vi "main_prototipo.vi"() -> ()   [LabVIEW 2021]
uses:
  Ctls/msg.ctl
  <vilib>/MakerHub/LINX/Private/Type Defs/LINX Ref.ctl
  <vilib>/MakerHub/LINX/Private/Type Defs/Platform.ctl
  <vilib>/MakerHub/LINX/Private/Type Defs/Interface.ctl
  <vilib>/MakerHub/LINX/Private/Device/Type Defs/LINX Device Config.ctl
  <vilib>/MakerHub/LINX/Private/Device/Type Defs/TCP Config.ctl
  <vilib>/MakerHub/LINX/Private/Device/Type Defs/Channels.ctl
  <vilib>/MakerHub/LINX/LMH-LINX.lvlib
  <vilib>/MakerHub/LINX/Private/Device/Device.lvlib
panel:
  in  "Stop":bool
  out "Datos Leídos":string[](array[string])
  in  "Buadrate":u32=8
  in  "Puerto COM":refnum<visa-resource-name>
  in  "TyP":bool
  out "Error Out 2":errorcluster
  in  "Error In 2":errorcluster
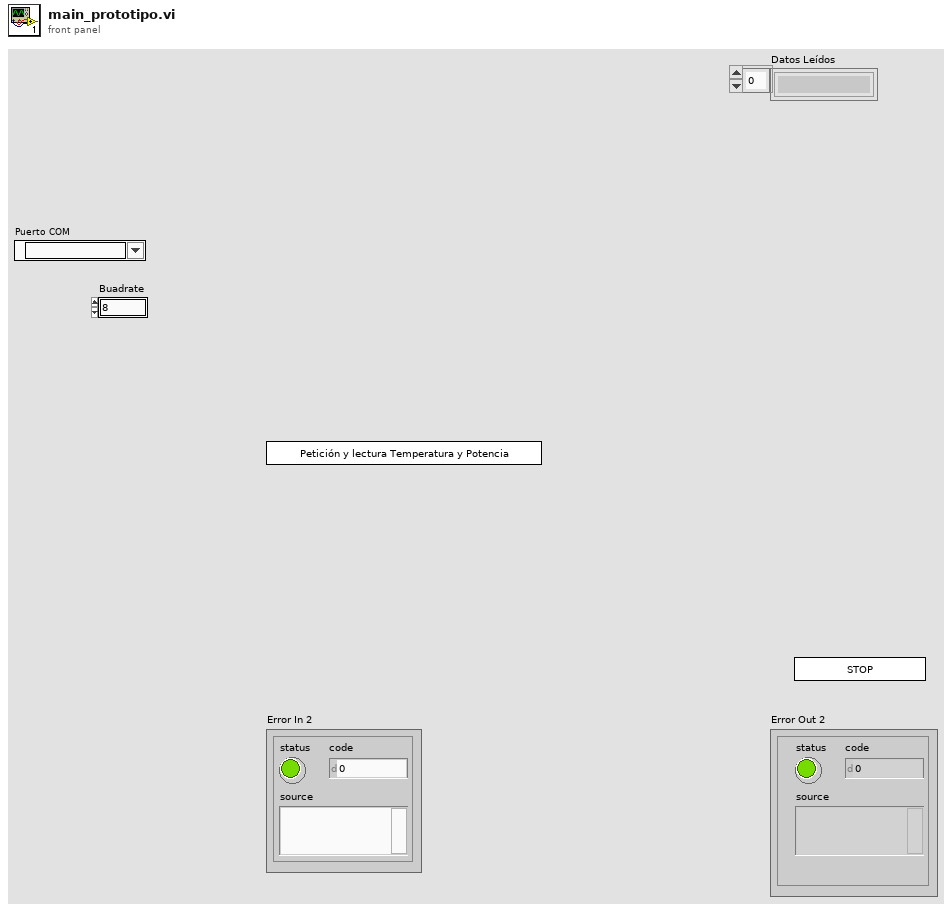
[diagram p1: front panel]
types:
  T1 = typedef "LMH-LINX.lvlib/LINX Ref.ctl" = cluster{"IO":T2, "Interface":T3, "LINX Device Config":T4}
  T2 = typedef "LMH-LINX.lvlib/Platform.ctl" = enum16{"Remote", "Local"}
  T3 = typedef "LMH-LINX.lvlib/Interface.ctl" = enum16{"Serial", "TCP"}
  T4 = typedef "LMH-LINX.lvlib/Device.lvlib/LINX Device Config.ctl" = cluster{"Interface":T3, "COM Port":refnum<visa-resource-name>, "TCP Configuration":T5, "Device Family":u8, "Device ID":u8, "Device Name":string, "TCP Ref":refnum<k5>, "Channels":T6}
  T5 = typedef "LMH-LINX.lvlib/Device.lvlib/TCP Config.ctl" = cluster{"IP Address":string, "Port":u16}
  T6 = typedef "LMH-LINX.lvlib/Channels.ctl" = cluster{"DI":u8[], "DO":u8[], "AI":u8[], "AO":u8[], "PWM":u8[], "QE":u8[], "UART":u8[], "I2C 2":u8[], "SPI":u8[], "CAN":u8[], "Servo":u8[], "AI Ref (V)":dbl, "AI Resolution (Bits)":u8, "AO Ref (V)":dbl, "AO Resolution (Bits)":u8}
  T7 = typedef "msg.ctl" = cluster{"mensaje":string, "info":cluster{"I2C Slave Address ":u8, "Data":u8[], "Bytes To Read":u8}, "LINX Resource":T1}
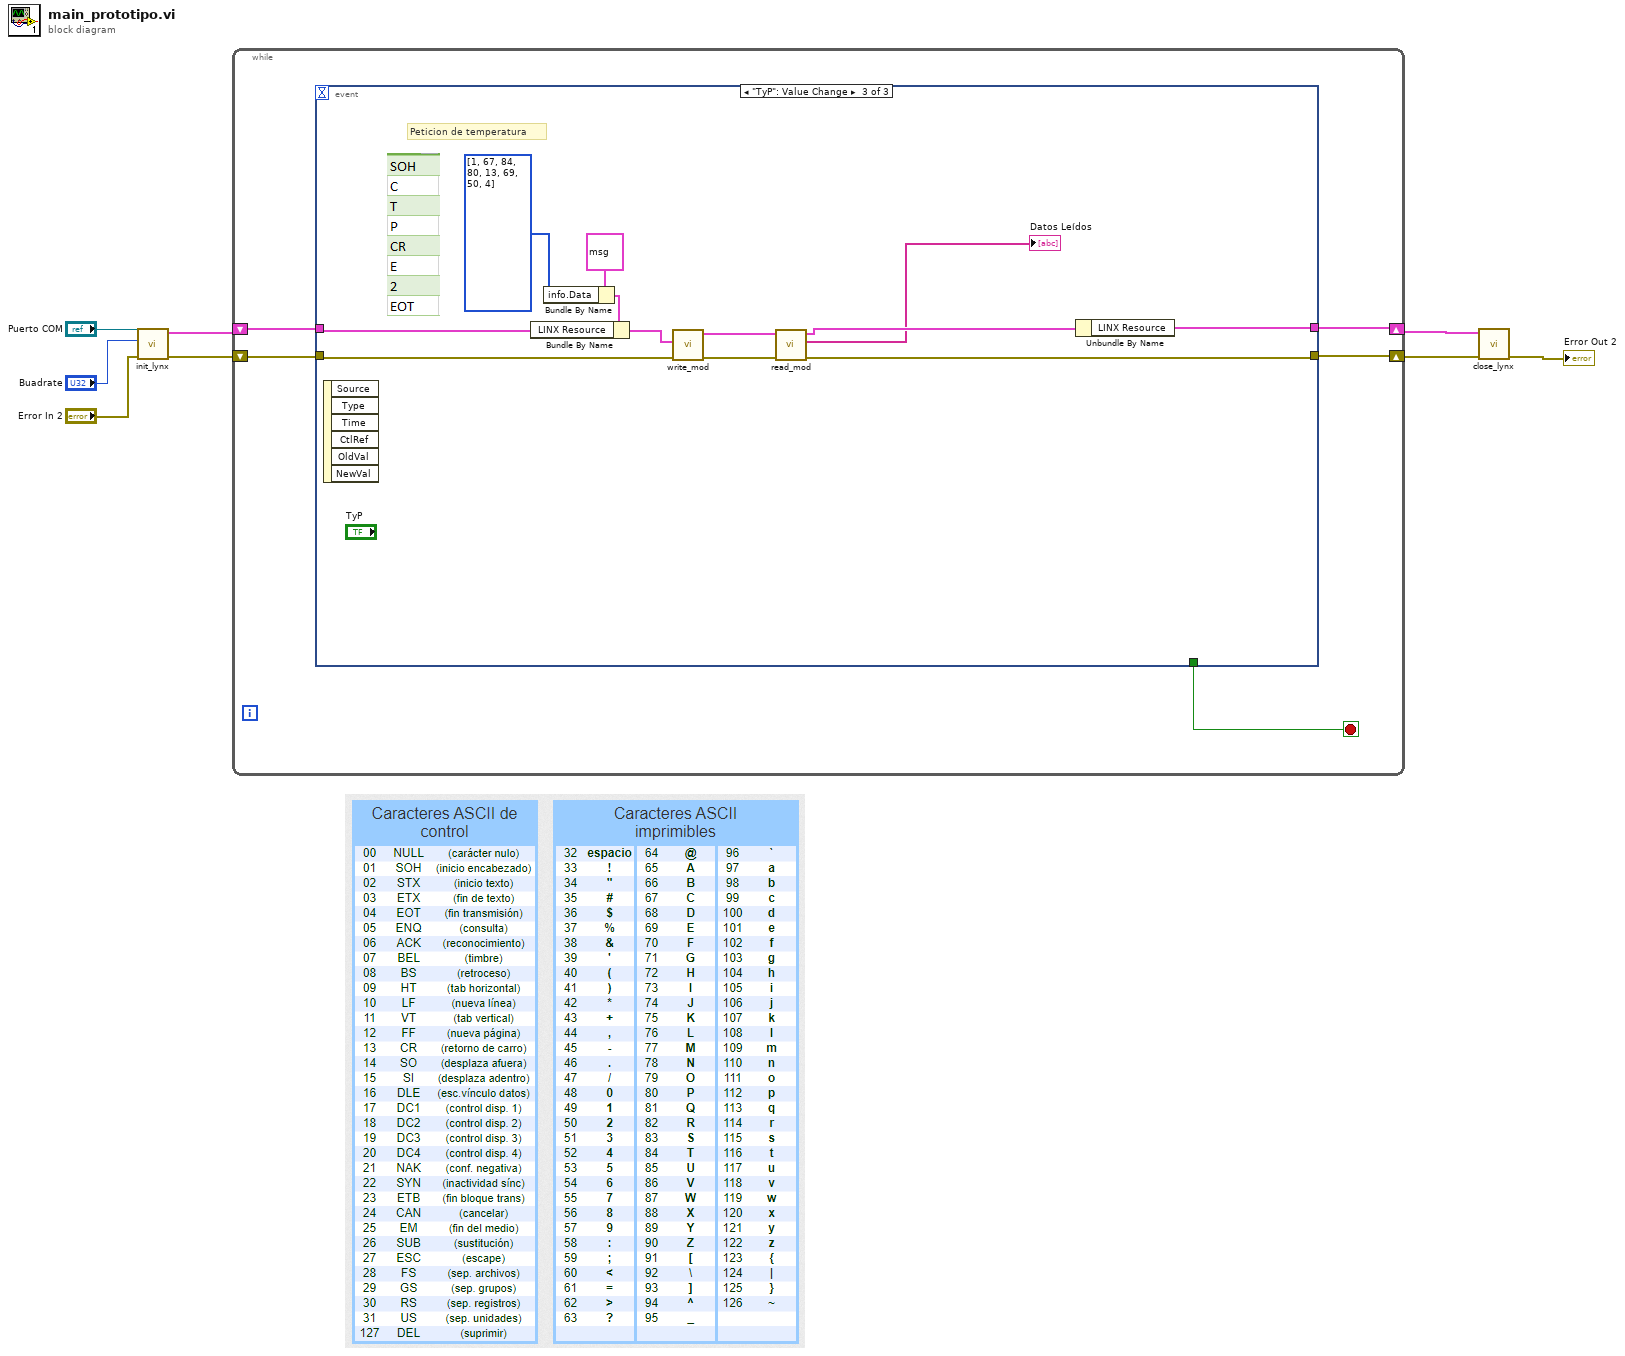
[diagram p0: block diagram]
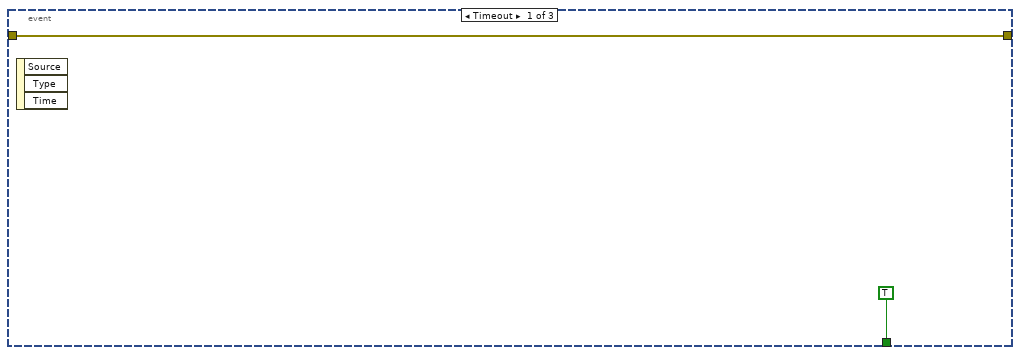
[diagram p2: hidden frame]
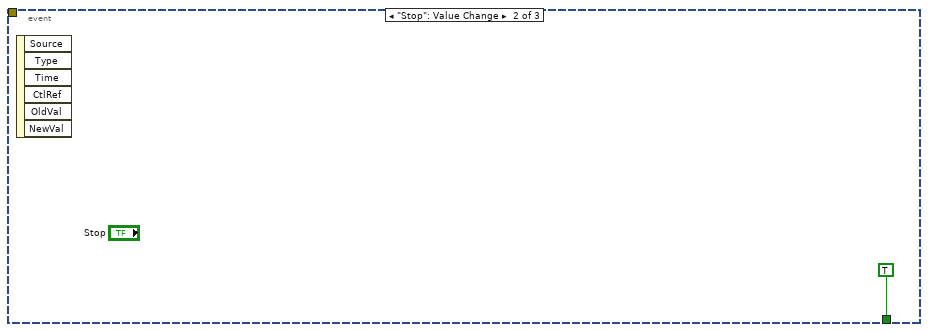
[diagram p3: hidden frame]
diagram:
  n1 = call "init_lynx.vi"("Error In 2"="Error In 2", "Baud Rate Override"="Buadrate", "Serial Port 2"="Puerto COM") -> ("Error Out"=w7:errorcluster, "LINX Resource"=w4:T1)  [unwired: 7 in]
  n2 = while {
    shift-right: [w11] -> w6
    shift-left: w7 -> [w12]
    shift-right: [w10] -> w3
    shift-left: w4 -> [w13]
    stop <- w9 stop-if-true
    n3 = event shown="[2] \"TyP\": Value Change" {
      selector: _ -> [_ _ _]
      dyn-events: _ -> [_ _ _]
      timeout: _ -> [_ _ _]
      tunnel: w13 -> [_ _ w23]
      tunnel: w12 -> [w15 _ w28]
      tunnel: [_ _ w24] -> w10
      tunnel: [w15 _ w26] -> w11
      tunnel: [TRUE ("Stop") TRUE ("Stop") _] -> w9
      event Timeout {
        n4 = event-data() -> ()  [unwired: 1 in, 3 out]
      }
      event "Stop": Value Change {
        n5 = event-data() -> ()  [unwired: 1 in, 6 out]
      }
      event "TyP": Value Change {
        # "Peticion de temperatura"
        n6 = event-data() -> ()  [unwired: 1 in, 6 out]
        n7 = Bundle By Name(cluster=T7 {"mensaje"="", "info"={"I2C Slave Address "=8, "Data"=[0], "Bytes To Read"=1}, "LINX Resource"={"IO"=enum."Remote", "Interface"=enum."Serial", "LINX Device Config"={"Interface"=enum."Serial", "COM Port"="COM4", "TCP Configuration"={"IP Address"="", "Port"=0}, "Device Family"=2, "Device ID"=0, "Device Name"="Arduino Uno\u0000", "TCP Ref"=refnum, "Channels"={"DI"=[0, 1, 2, 3, 4, 5, 6, 7, 8, 9, 10, 11, 12, 13, 14, 15, 16, 17, 18, 19], "DO"=[0, 1, 2, 3, 4, 5, 6, 7, 8, 9, 10, 11, 12, 13, 14, 15, 16, 17, 18, 19], "AI"=[0, 1, 2, 3, 4, 5], "AO"=[], "PWM"=[3, 5, 6, 9, 10, 11], "QE"=[], "UART"=[0], "I2C 2"=[0], "SPI"=[0], "CAN"=[], "Servo"=[0, 1, 2, 3, 4, 5, 6, 7, 8, 9, 10, 11, 12, 13, 14, 15, 16, 17, 18, 19], "AI Ref (V)"=5.0, "AI Resolution (Bits)"=0, "AO Ref (V)"=0.0, "AO Resolution (Bits)"=0}}}} ("msg"), "info.Data"=u8[] [1, 67, 84, 80, 13, 69, 50, 4]) -> (w17:T7)
        n8 = Bundle By Name(cluster=w17, "LINX Resource"=w23) -> (w22:T7)
        n9 = call "write_mod.vi"("error in (no error)"=w28, "msg"=w22) -> ("error out"=w27:errorcluster, "msg 3"=w21:T7)  [unwired: 8 in]
        n10 = call "read_mod.vi"("error in (no error)"=w27, "msg"=w21) -> ("error out"=w26:errorcluster, "Datos Leídos"=→"Datos Leídos":string[], "output cluster"=w25:T7)  [unwired: 6 in, 1 out]
        n11 = Unbundle By Name(w25) -> ("LINX Resource"=w24:T1)
      }
    }
  }
  n12 = call "close_lynx.vi"("Error In"=w6, "LINX Resource"=w3) -> ("Error Out 2"=→"Error Out 2":errorcluster)  [unwired: 9 in]
